vi "Disable All Buttons_UI.vi"(8 "error in (no error)":errorcluster, 10 "state":string, 11 "ZenGage v3.0 UI in":T1) -> (0 "error out":errorcluster)   [LabVIEW 2019, in "ZenGage v3.0 UI.lvclass"]
uses:
  ZenGage v3.0 UI.lvclass
  Type Definitions/Controls and Indicators/Select a part (combobox).ctl
  Type Definitions/Controls and Indicators/EDL control references.ctl
  Type Definitions/Controls and Indicators/Diagnostics control referencs.ctl
  Type Definitions/Controls and Indicators/Inspection control references.ctl
  Type Definitions/Controls and Indicators/General_Control references.ctl
  Type Definitions/Controls and Indicators/Controls and Indicators Cluster.ctl
  Type Definitions/General/Master sample references.ctl
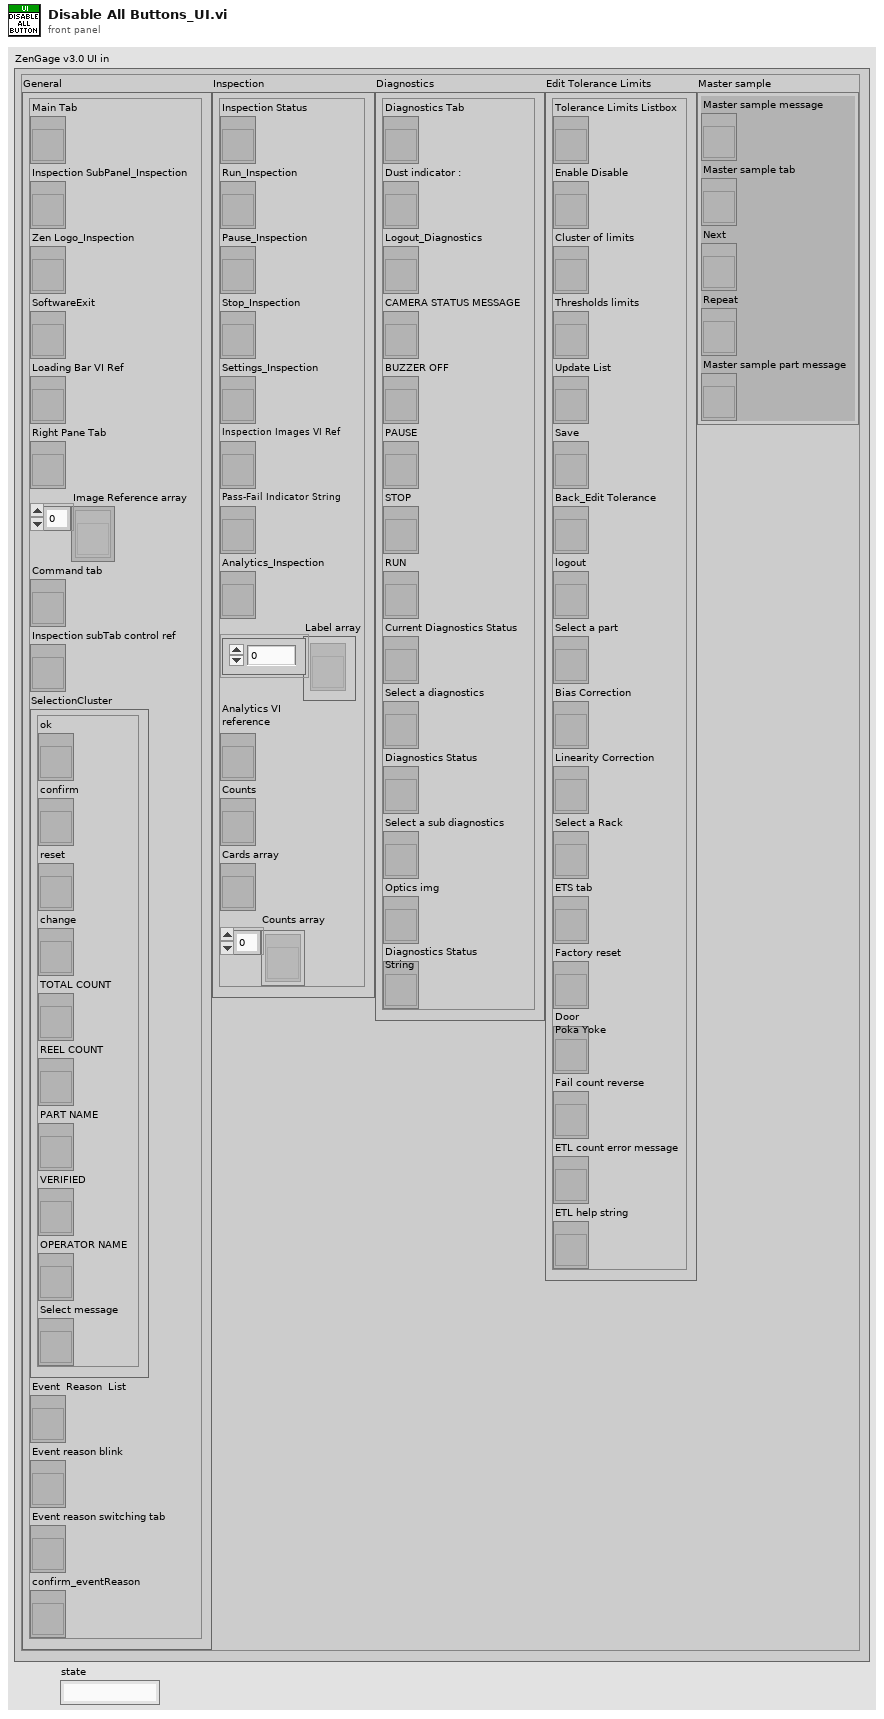
[diagram p1: front panel]
types:
  T1 = typedef "ZenGage v3.0 UI.lvclass/Controls and Indicators Cluster.ctl" = cluster{"General":T2, "Inspection":T3, "Diagnostics":T4, "Edit Tolerance Limits":T5, "Master sample":T6}
  T2 = typedef "ZenGage v3.0 UI.lvclass/General_Control references.ctl" = cluster{"Main Tab":refnum<vi>, "Inspection SubPanel_Inspection":refnum<vi>, "Zen Logo_Inspection":refnum<vi>, "SoftwareExit":refnum<vi>, "Loading Bar VI Ref":refnum<vi>, "Right Pane Tab":refnum<vi>, "Image Reference array":refnum<vi>[], "Command tab":refnum<vi>, "Inspection subTab control ref":refnum<vi>, "SelectionCluster":cluster{"ok":refnum<vi>, "confirm":refnum<vi>, "reset":refnum<vi>, "change":refnum<vi>, "TOTAL COUNT":refnum<vi>, "REEL COUNT":refnum<vi>, "PART NAME":refnum<vi>, "VERIFIED":refnum<vi>, "OPERATOR NAME":refnum<vi>, "Select message":refnum<vi>}, "Event  Reason  List":refnum<vi>, "Event reason blink":refnum<vi>, "Event reason switching tab":refnum<vi>, "confirm_eventReason":refnum<vi>}
  T3 = typedef "ZenGage v3.0 UI.lvclass/Inspection control references.ctl" = cluster{"Inspection Status":refnum<vi>, "Run_Inspection":refnum<vi>, "Pause_Inspection":refnum<vi>, "Stop_Inspection":refnum<vi>, "Settings_Inspection":refnum<vi>, "Inspection Images VI Ref":refnum<vi>, "Pass-Fail Indicator String":refnum<vi>, "Analytics_Inspection":refnum<vi>, "Label array":refnum<vi>[], "Analytics VI\nreference":refnum<vi>, "Counts":refnum<vi>, "Cards array":refnum<vi>, "Counts array":refnum<vi>[]}
  T4 = typedef "ZenGage v3.0 UI.lvclass/Diagnostics control referencs.ctl" = cluster{"Diagnostics Tab":refnum<vi>, "Dust indicator :":refnum<vi>, "Logout_Diagnostics":refnum<vi>, "CAMERA STATUS MESSAGE":refnum<vi>, "BUZZER OFF":refnum<vi>, "PAUSE":refnum<vi>, "STOP":refnum<vi>, "RUN":refnum<vi>, "Current Diagnostics Status":refnum<vi>, "Select a diagnostics":refnum<vi>, "Diagnostics Status":refnum<vi>, "Select a sub diagnostics":refnum<vi>, "Optics img":refnum<vi>, "Diagnostics Status\nString":refnum<vi>}
  T5 = typedef "ZenGage v3.0 UI.lvclass/EDL control references.ctl" = cluster{"Tolerance Limits Listbox":refnum<vi>, "Enable Disable":refnum<vi>, "Cluster of limits":refnum<vi>, "Thresholds limits":refnum<vi>, "Update List":refnum<vi>, "Save":refnum<vi>, "Back_Edit Tolerance":refnum<vi>, "logout":refnum<vi>, "Select a part":refnum<vi>, "Bias Correction":refnum<vi>, "Linearity Correction":refnum<vi>, "Select a Rack":refnum<vi>, "ETS tab":refnum<vi>, "Factory reset":refnum<vi>, "Door\nPoka Yoke":refnum<vi>, "Fail count reverse":refnum<vi>, "ETL count error message":refnum<vi>, "ETL help string":refnum<vi>}
  T6 = typedef "Master sample references.ctl" = cluster{"Master sample message":refnum<vi>, "Master sample tab":refnum<vi>, "Next":refnum<vi>, "Repeat":refnum<vi>, "Master sample part message":refnum<vi>}
  T7 = enum8{"Enabled", "Disabled", "Disabled and Grayed Out"}
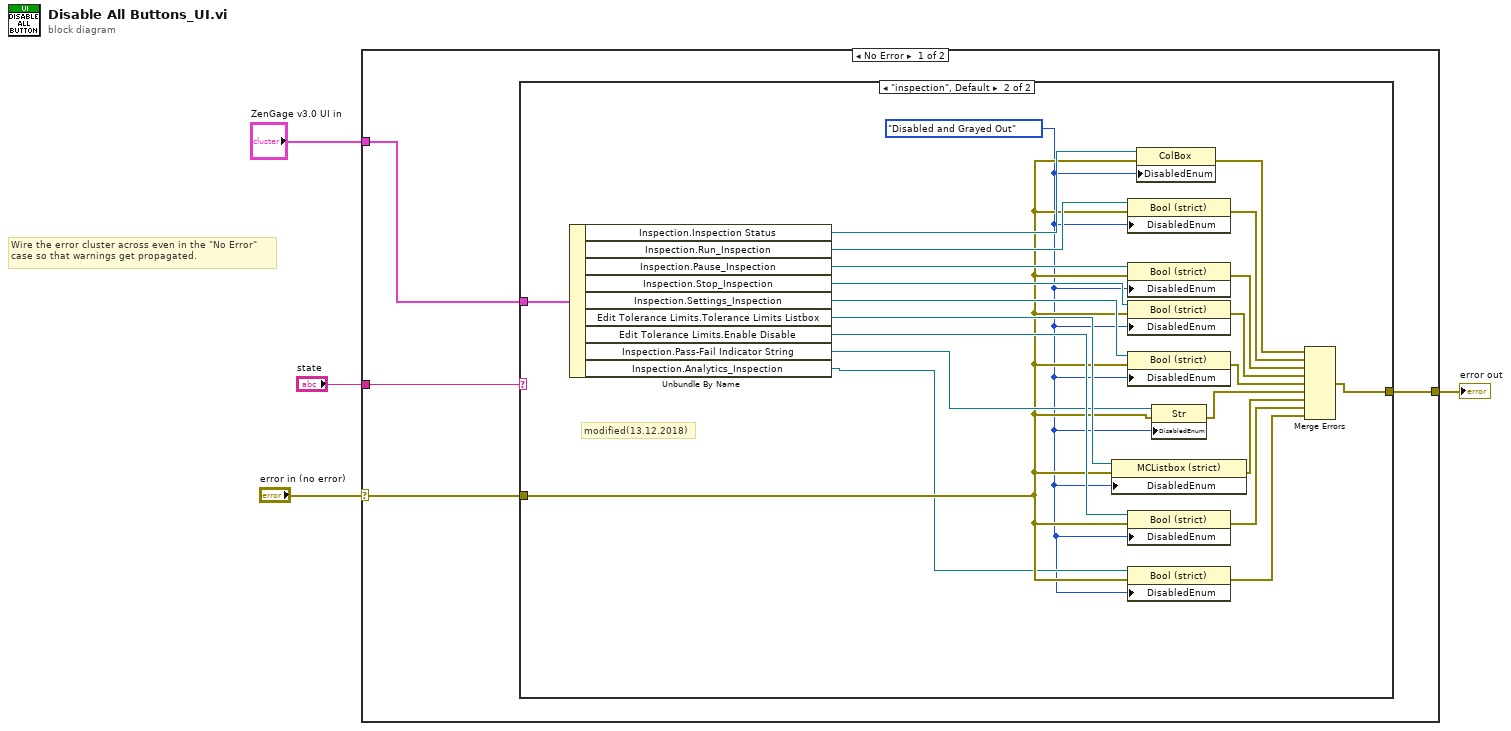
[diagram p0: block diagram]
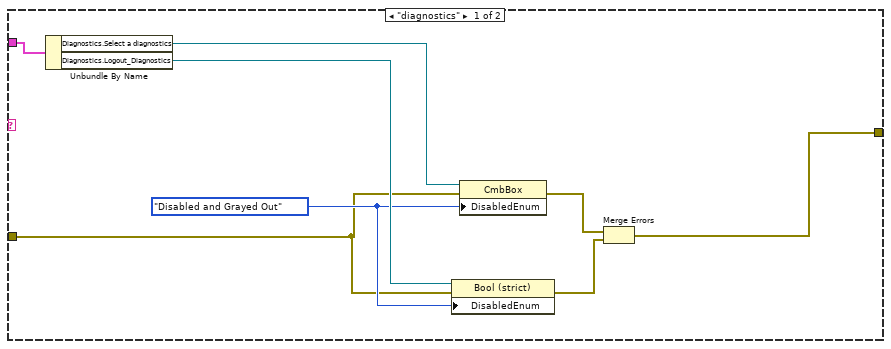
[diagram p2: hidden frame]
diagram:
  # "Wire the error cluster across even in the \"No Error\"\ncase so that warnings get propagated."
  n1 = case shown="No Error" "error in (no error)" {
    selector: "error in (no error)" -> [w6 w39]
    tunnel: [w7 w39] -> w3
    tunnel: "ZenGage v3.0 UI in" -> [w8 _]
    tunnel: "state" -> [w5 _]
    frame No Error {
      n2 = case shown="\"inspection\", Default" w5 {
        tunnel: w8 -> [w16 w38]
        tunnel: [w11 w23] -> w7
        tunnel: w6 -> [w9 w20]
        frame "diagnostics" {
          w13 = T7."Disabled and Grayed Out" ("Disabled")
          n3 = Unbundle By Name(w16) -> ("Diagnostics.Select a diagnostics"=w15:refnum<vi>, "Diagnostics.Logout_Diagnostics"=w14:refnum<vi>)
          n4 = property class="Bool (strict)"(reference=w14, error in=w9, "DisabledEnum"=w13) -> (error out=w10:errorcluster)  [unwired: 1 out]
          n5 = property class="CmbBox"(reference=w15, error in=w9, "DisabledEnum"=w13) -> (error out=w12:errorcluster)  [unwired: 1 out]
          n6 = Merge Errors(w12, w10) -> (w11:errorcluster)
        }
        frame "inspection", Default {
          w17 = T7."Disabled and Grayed Out" ("Disabled")
          # "modified(13.12.2018)"
          n7 = Unbundle By Name(w38) -> ("Inspection.Inspection Status"=w37:refnum<vi>, "Inspection.Run_Inspection"=w36:refnum<vi>, "Inspection.Pause_Inspection"=w35:refnum<vi>, "Inspection.Stop_Inspection"=w34:refnum<vi>, "Inspection.Settings_Inspection"=w33:refnum<vi>, "Edit Tolerance Limits.Tolerance Limits Listbox"=w32:refnum<vi>, "Edit Tolerance Limits.Enable Disable"=w31:refnum<vi>, "Inspection.Pass-Fail Indicator String"=w22:refnum<vi>, "Inspection.Analytics_Inspection"=w19:refnum<vi>)
          n8 = property class="MCListbox (strict)"(reference=w32, error in=w20, "DisabledEnum"=w17) -> (error out=w25:errorcluster)  [unwired: 1 out]
          n9 = property class="Bool (strict)"(reference=w36, error in=w20, "DisabledEnum"=w17) -> (error out=w29:errorcluster)  [unwired: 1 out]
          n10 = property class="Bool (strict)"(reference=w35, error in=w20, "DisabledEnum"=w17) -> (error out=w28:errorcluster)  [unwired: 1 out]
          n11 = property class="Bool (strict)"(reference=w34, error in=w20, "DisabledEnum"=w17) -> (error out=w27:errorcluster)  [unwired: 1 out]
          n12 = property class="Bool (strict)"(reference=w33, error in=w20, "DisabledEnum"=w17) -> (error out=w26:errorcluster)  [unwired: 1 out]
          n13 = property class="Bool (strict)"(reference=w31, error in=w20, "DisabledEnum"=w17) -> (error out=w24:errorcluster)  [unwired: 1 out]
          n14 = property class="Bool (strict)"(reference=w19, error in=w20, "DisabledEnum"=w17) -> (error out=w18:errorcluster)  [unwired: 1 out]
          n15 = property class="ColBox"(reference=w37, error in=w20, "DisabledEnum"=w17) -> (error out=w30:errorcluster)  [unwired: 1 out]
          n16 = property class="Str"(reference=w22, error in=w20, "DisabledEnum"=w17) -> (error out=w21:errorcluster)  [unwired: 1 out]
          n17 = Merge Errors(w30, w29, w28, w27, w26, w21, w25, w24, w18) -> (w23:errorcluster)
        }
      }
    }
    frame Error {
    }
  }
  "error out" <- w3
